vi "Médias.vi"(1 "Infos para processamento":T1={"Diâmetro do furo [mm]"=1.4, "Diâmetro da linha média [mm]"=5.0, "IncF"=0.2, "Módulo de elasticidade [GPa]"=207.0, "Módulo de Poisson"=0.3, "Tipo de roseta utilizada"=enum."Tipo A", "Método de análise"=enum."Simplificado 2008", "Pfinal"=0.3, "Parar auto."=TRUE}, 2 "Dados":string) -> (0 "Dados":T2)   [LabVIEW 2016]
uses:
  Controles/Infos para processamento.ctl
  <vilib>/Analysis/1siggen.llb/Ramp Pattern by Samples.vi
  <vilib>/Analysis/baseanly.llb/Mean (DBL).vi
  <vilib>/Analysis/NI_AALBase.lvlib
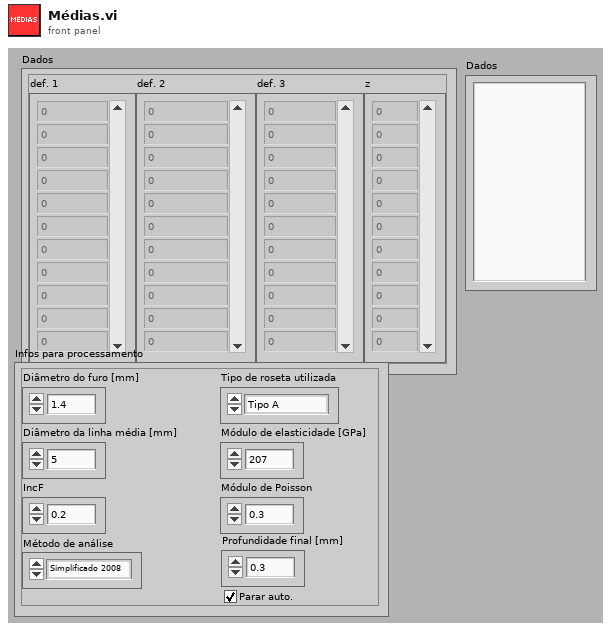
[diagram p1: front panel]
types:
  T1 = typedef "Infos para processamento.ctl" = cluster{"Diâmetro do furo [mm]":dbl, "Diâmetro da linha média [mm]":dbl, "IncF":dbl, "Módulo de elasticidade [GPa]":dbl, "Módulo de Poisson":dbl, "Tipo de roseta utilizada":enum16{"Tipo A", "Tipo B", "Tipo C"}, "Método de análise":enum16{"Não uniforme 2013", "Simplificado 2013", "Simplificado 2008"}, "Pfinal":dbl, "Parar auto.":bool}
  T2 = typedef "Deformações.ctl" = cluster{"def. 1 ":dbl[], "def. 2":dbl[], "def. 3":dbl[], "z":dbl[]}
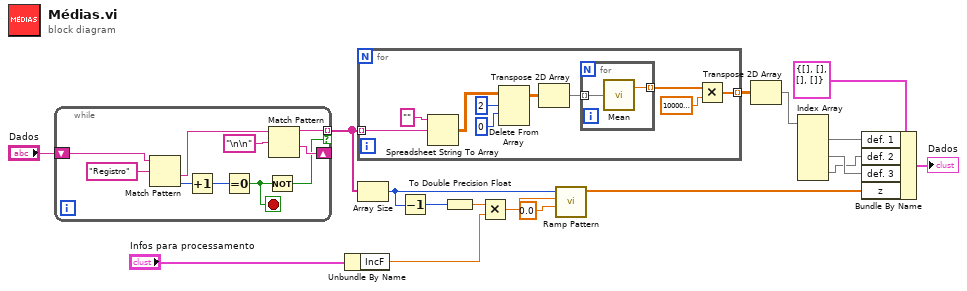
[diagram p0: block diagram]
diagram:
  n1 = while {
    shift-right: [w22] -> _
    shift-left: "Dados" -> [w27]
    tunnel: [w23] -> w4 mode=indexing if=w18
    stop <- w19 stop-if-true
    n2 = Match Pattern(string=w27, regular expression="Registro") -> (after substring=w25:string, offset past match=w21:i32)  [unwired: 1 in, 2 out]
    n3 = Increment(x=w21) -> (x+1=w20:i32)
    n4 = Equal To 0?(x=w20) -> (x = 0?=w19:bool)
    n5 = Not(x=w19) -> (.not. x?=w18:bool)
    n6 = Match Pattern(string=w25, regular expression="\n\n") -> (before substring=w23:string, after substring=w22:string)  [unwired: 1 in, 2 out]
  }
  n7 = Unbundle By Name("Infos para processamento") -> ("IncF"=w6:dbl)
  n8 = for {
    tunnel: w4 -> [w37] mode=indexing
    tunnel: [w28] -> w5 mode=indexing
    n9 = Spreadsheet String To Array(format string="", spreadsheet string=w37) -> (array=w35:dbl[][])  [unwired: 2 in]
    n10 = Delete From Array(array=w35, length=2, index (row)=0) -> (array with subset deleted=w32:dbl[][])  [unwired: 1 in, 1 out]
    n11 = Transpose 2D Array(2D array=w32) -> (transposed array=w31:dbl[][])
    n12 = for {
      tunnel: w31 -> [w39] mode=indexing
      tunnel: [w38] -> w30 mode=indexing
      n13 = call-poly <vilib>:"Mean.vi"("X"=w39) -> ("mean"=w38:dbl)  [unwired: 1 out]
    }
    n14 = Multiply(x=w30, y=1000000.0 ("Profundidade inicial [mm]:")) -> (x*y=w28:dbl[])
  }
  n15 = Array Size(array=w4) -> (size(s)=w3:i32)
  n16 = Decrement(x=w3) -> (x-1=w8:i32)
  n17 = To Double Precision Float(number=w8) -> (double precision float=w16:dbl)
  n18 = Multiply(x=w16, y=w6) -> (x*y=w15:dbl)
  n19 = call-poly <vilib>:"Ramp Pattern.vi"("start"=0.0 ("Profundidade inicial [mm]:"), "end"=w15, "samples"=w3) -> ("Ramp Pattern"=w12:dbl[])  [unwired: 7 in, 1 out]
  n20 = Transpose 2D Array(2D array=w5) -> (transposed array=w9:dbl[][])
  n21 = Index Array(array=w9) -> (element #1=w11:dbl[], element #2=w2:dbl[], element #3=w1:dbl[])  [unwired: 6 in]
  n22 = Bundle By Name(cluster=T2 {"def. 1 "=[], "def. 2"=[], "def. 3"=[], "z"=[]} ("Dados"), "def. 1"=w11, "def. 2"=w1, "def. 3"=w2, "z"=w12) -> (→"Dados":T2)
